vi "4x7 Example Implementation.vi"() -> ()   [LabVIEW 2022 SP3]
uses:
  <vilib>/MakerHub/LINX/Public/Utilities/Open Serial.vi
  <vilib>/MakerHub/LINX/LMH-LINX.lvlib
panel:
  in  "Combo":i32=4
  in  "stop":bool
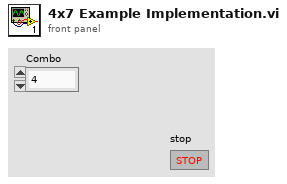
[diagram p1: front panel]
types:
  T1 = typedef "LMH-LINX.lvlib/LINX Ref.ctl" = cluster{"IO":T2, "Interface":T3, "LINX Device Config":T4}
  T2 = typedef "LMH-LINX.lvlib/Platform.ctl" = enum16{"Remote", "Local"}
  T3 = typedef "LMH-LINX.lvlib/Interface.ctl" = enum16{"Serial", "TCP"}
  T4 = typedef "LMH-LINX.lvlib/Device.lvlib/LINX Device Config.ctl" = cluster{"Interface":T3, "COM Port":refnum<visa-resource-name>, "TCP Configuration":T5, "Device Family":u8, "Device ID":u8, "Device Name":string, "TCP Ref":refnum<k5>, "Channels":T6}
  T5 = typedef "LMH-LINX.lvlib/Device.lvlib/TCP Config.ctl" = cluster{"IP Address":string, "Port":u16}
  T6 = typedef "LMH-LINX.lvlib/Channels.ctl" = cluster{"DI":u8[], "DO":u8[], "AI":u8[], "AO":u8[], "PWM":u8[], "QE":u8[], "UART":u8[], "I2C 2":u8[], "SPI":u8[], "CAN":u8[], "Servo":u8[], "AI Ref (V)":dbl, "AI Resolution (Bits)":u8, "AO Ref (V)":dbl, "AO Resolution (Bits)":u8}
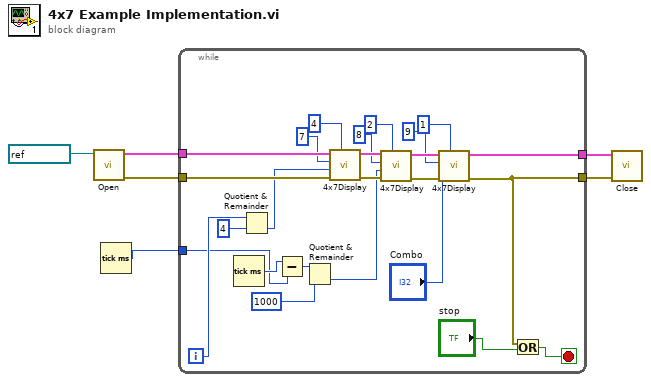
[diagram p0: block diagram]
diagram:
  n1 = call-poly <vilib>:"Open.vi"("Serial Port"=refnum<visa-resource-name> "COM4") -> ("Error Out"=w3:errorcluster, "LINX Resource"=w6:T1)  [unwired: 8 in, 1 out]
  n2 = Tick Count (ms)() -> (millisecond timer value=w1:u32)
  n3 = while {
    tunnel: w6 -> [w29]
    tunnel: [w11] -> w5
    tunnel: [w10] -> w4
    tunnel: w3 -> [w28]
    tunnel: w1 -> [w16]
    i -> [w26]
    stop <- w31 stop-if-true
    n4 = Tick Count (ms)() -> (millisecond timer value=w17:u32)
    n5 = Quotient & Remainder(x=w26, y=4) -> (floor(x/y)=w21:i32)  [unwired: 1 out]
    n6 = Subtract(x=w17, y=w16) -> (x-y=w18:u32)
    n7 = Quotient & Remainder(x=w18, y=1000) -> (floor(x/y)=w19:u32)  [unwired: 1 out]
    n8 = call "4x7Display.vi"("Display Length"=4, "Error In"=w28, "Input"=w21, "Custom Command Number"=u16 7, "LINX Resource In"=w29) -> ("Error Out"=w23:errorcluster, "LINX Resource Out"=w24:T1)  [unwired: 5 in]
    n9 = call "4x7Display.vi"("Display Length"=2, "Error In"=w23, "Input"=w19, "Custom Command Number"=u16 8, "LINX Resource In"=w24) -> ("Error Out"=w13:errorcluster, "LINX Resource Out"=w12:T1)  [unwired: 5 in]
    n10 = call "4x7Display.vi"("Display Length"=1, "Error In"=w13, "Input"="Combo", "Custom Command Number"=u16 9, "LINX Resource In"=w12) -> ("Error Out"=w10:errorcluster, "LINX Resource Out"=w11:T1)  [unwired: 5 in]
    n11 = Or(x=w10, y="stop") -> (x .or. y?=w31:bool)
  }
  n12 = call <vilib>:"Close.vi"("Error In"=w4, "LINX Resource"=w5) -> ()  [unwired: 9 in, 1 out]
